vi "Parse-command-line-arguments.vi"(8 "error in (no error)":errorcluster, 9 "Client channel in":refnum<queue>, 10 "Server channel in":refnum<queue>) -> (0 "error out":errorcluster, 1 "Client channel":refnum<queue>, 2 "Server channel":refnum<queue>)   [LabVIEW 2013, in "SLMControl.lvlib" / "SC-Main.lvclass"]
uses:
  SC-Main.lvclass
  SA-SLMAPI/Sources/Message.lvclass
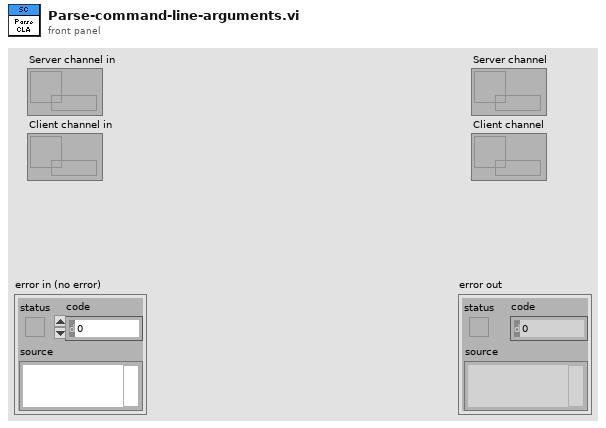
[diagram p1: front panel]
types:
  T1 = enum32{"invalid app kind", "Development System", "Run Time System", "Student Edition", "Embedded LabVIEW", "Evaluation", "Custom"}
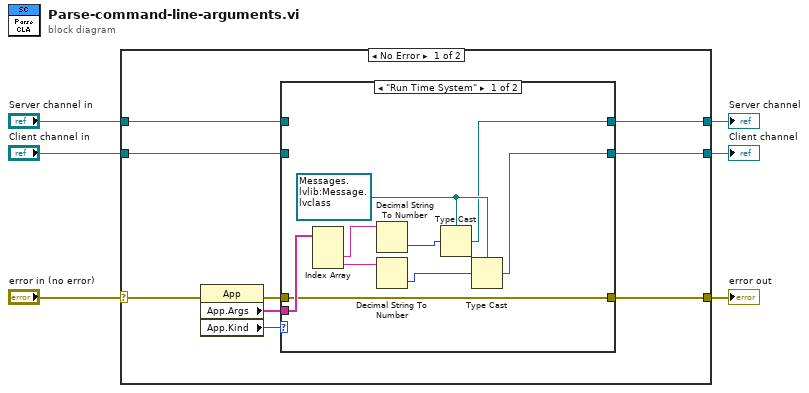
[diagram p0: block diagram]
diagram:
  n1 = case shown="No Error" "error in (no error)" {
    selector: "error in (no error)" -> [w12 w30]
    tunnel: [w11 w30] -> w5
    tunnel: "Server channel in" -> [w10 w29]
    tunnel: "Client channel in" -> [w9 w28]
    tunnel: [w8 w29] -> w2
    tunnel: [w7 w28] -> w1
    frame No Error {
      n2 = property class="App"(error in=w12) -> (error out=w14:errorcluster, "App.Args"=w13:string[], "App.Kind"=w15:T1)  [unwired: 1 in, 1 out]
      n3 = case shown="\"Run Time System\"" w15 {
        tunnel: w14 -> [w23 w27]
        tunnel: [w23 w27] -> w11
        tunnel: w13 -> [w24 _]
        tunnel: w10 -> [_ w26]
        tunnel: w9 -> [_ w25]
        tunnel: [w16 w26] -> w8
        tunnel: [w19 w25] -> w7
        frame "Run Time System" {
          w17 = refnum<queue> refnum ("Com-out")
          n4 = Index Array(array=w24) -> (element #2=w21:string, element #3=w22:string)  [unwired: 3 in, 1 out]
          n5 = Decimal String To Number(string=w21) -> (number=w18:i32)  [unwired: 2 in, 1 out]
          n6 = Decimal String To Number(string=w22) -> (number=w20:i32)  [unwired: 2 in, 1 out]
          n7 = Type Cast(type=w17, x=w18) -> (*(type *) &x=w16:refnum<queue>)
          n8 = Type Cast(type=w17, x=w20) -> (*(type *) &x=w19:refnum<queue>)
        }
        frame Default {
        }
      }
    }
    frame Error {
    }
  }
  "error out" <- w5
  "Server channel" <- w2
  "Client channel" <- w1
